vi "Drive Control Global.vi"() -> ()   [LabVIEW 2009]
panel:
  in  "# of ticks/count recorded":i32
  in  "Drive Encoder tick/count":u32
  in  "Drive Encoder ft/sec":fxp<+/-,18,8>
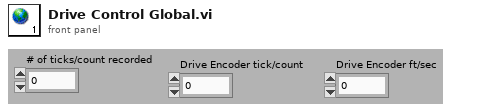
[diagram p1: front panel]
diagram:
